vi "SingleCounter - Arm.vi"(4 "Duration":dbl=20000000.0, 5 "Trigger Source":tag="/Dev1/PFI33", 6 "CI.Prescaler":u32, 7 "Sampling Rate":dbl=20000000.0, 8 "Error In":errorcluster, 9 "Clock Source":tag="/Dev1/20MHzTimebase", 10 "External Timing Source":tag="/Dev1/PFI39", 11 "counter":tag="Dev1/ctr0") -> (0 "error out":errorcluster, 3 "task out":refnum<k21>)   [LabVIEW 2018]
uses:
  <vilib>/DAQmx/create/channels.llb/DAQmx Create Channel (CI-Count Edges).vi
  <vilib>/DAQmx/configure/timing.llb/DAQmx Timing (Sample Clock).vi
  <resource>/objmgr/daqmx.rc
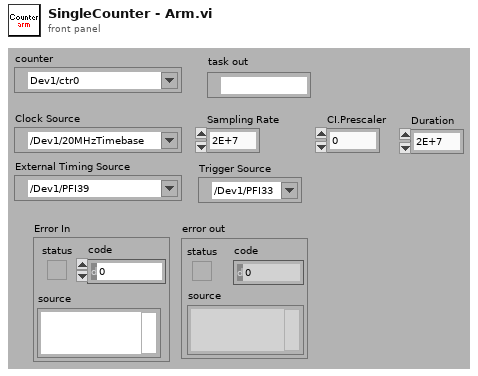
[diagram p1: front panel]
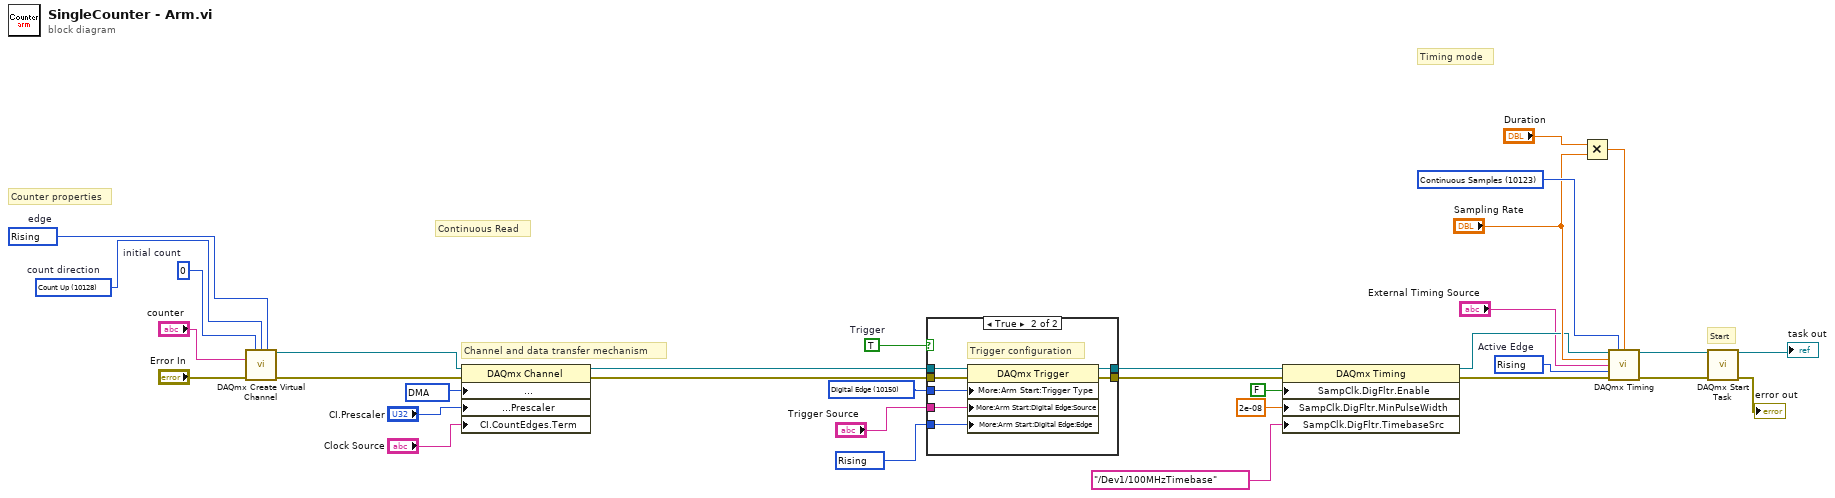
[diagram p0: block diagram]
diagram:
  w30 = 10280 items=["Rising"=10280, "Falling"=10171] ("Trigger Edge")
  w31 = 10150 items=["Digital Edge"=10150, "None"=10230] ("Trigger Type")
  w32 = TRUE  # Trigger
  w29 = 10280 items=["Rising"=10280, "Falling"=10171]  # Active Edge
  w26 = 10128 items=["Count Up"=10128, "Count Down"=10124, "Externally Controlled"=10326]  # count direction
  w27 = 10280 items=["Rising"=10280, "Falling"=10171]  # edge
  w21 = u32 0  # initial count
  w20 = 10054 items=["DMA"=10054, "Interrupts"=10204, "Programmed I/O"=10264] ("CI.DataXferMech")
  w19 = 10123 items=["Finite Samples"=10178, "Continuous Samples"=10123, "Hardware Timed Single Point"=12522] ("Sample Mode")
  # "Continuous Read"
  # "Counter properties"
  # "Channel and data transfer mechanism"
  # "Timing mode"
  # "Start"
  n1 = call-poly <vilib>:"DAQmx Create Virtual Channel.vi"("initial count"=w21, "count direction"=w26, "edge"=w27, "counter"="counter", "error in"="Error In") -> ("task out"=w25:refnum<k21>, "error out"=w24:errorcluster)  [unwired: 9 in]
  n2 = property class="DAQmx Channel"(reference=w25, error in=w24, "Counter Input:General Properties:More:Advanced:Data Transfer and Memory:Data Transfer Mechanism"=w20, "Counter Input:General Properties:More:Advanced:Prescaler"="CI.Prescaler", "CI.CountEdges.Term"="Clock Source") -> (reference out=w3:refnum<k21>, error out=w2:errorcluster)
  n3 = case shown="True" w32 {
    tunnel: w3 -> [w35 w42]
    tunnel: w2 -> [w34 w41]
    tunnel: [w35 w40] -> w11
    tunnel: [w34 w39] -> w8
    tunnel: w31 -> [_ w38]
    tunnel: "Trigger Source" -> [_ w37]
    tunnel: w30 -> [_ w36]
    frame False {
    }
    frame True {
      # "Trigger configuration"
      n4 = property class="DAQmx Trigger"(reference=w42, error in=w41, "More:Arm Start:Trigger Type"=w38, "More:Arm Start:Digital Edge:Source"=w37, "More:Arm Start:Digital Edge:Edge"=w36) -> (reference out=w40:refnum<k21>, error out=w39:errorcluster)
    }
  }
  n5 = property class="DAQmx Timing"(reference=w11, error in=w8, "SampClk.DigFltr.Enable"=FALSE, "SampClk.DigFltr.MinPulseWidth"=2e-08, "SampClk.DigFltr.TimebaseSrc"=tag "/Dev1/100MHzTimebase") -> (reference out=w10:refnum<k21>, error out=w9:errorcluster)
  n6 = Multiply(x="Duration", y="Sampling Rate") -> (x*y=w14:dbl)
  n7 = call-poly <vilib>:"DAQmx Timing.vi"("task/channels in"=w10, "sample mode"=w19, "samples per channel"=w14, "rate"="Sampling Rate", "source"="External Timing Source", "active edge"=w29, "error in"=w9) -> ("task out"=w22:refnum<k21>, "error out"=w23:errorcluster)  [unwired: 7 in]
  n8 = call <vilib>:"DAQmx Start Task.vi"("task/channels in"=w22, "error in"=w23) -> ("task out"=→"task out":refnum<k21>, "error out"=→"error out":errorcluster)  [unwired: 12 in]
